vi "Actor Core.vi"(8 "error in":errorcluster, 11 "MakePrintTable in":refnum<class "MakePrintTable.lvclass">) -> (0 "error out":errorcluster, 3 "Actor out":refnum<class "Actor.lvclass">)   [LabVIEW 2015, in "ActorManagement.lvlib" / "MakePrintTable.lvclass"]
doc: "(<B>Filename</B>: Actor Framework.lvlib:Actor.lvclass:Actor Core.vi)\n\nReceives messages to the actor, reacts to them, and initiates any error handling that may shut the actor down.\n\nDescendant classes may override this VI to append parallel tasks for the actor to complete while it handles messages. Overrides use the Call Parent Method node."
uses:
  MakePrintTable.lvclass
  <vilib>/ActorFramework/Actor/Actor.lvclass
  <vilib>/ActorFramework/Actor/Actor.lvclass/Actor.ctl
  <vilib>/ActorFramework/Message Enqueuer/Message Enqueuer.lvclass/Message Enqueuer.ctl
  <vilib>/ActorFramework/Stop Msg/Stop Msg.lvclass/Stop Msg.ctl
  <vilib>/ActorFramework/Message Enqueuer/Init from Existing Queue.vi
  <vilib>/ActorFramework/Message Enqueuer/Enqueue Critical.vi
  <vilib>/ActorFramework/Message Priority Queue/Priority Enqueue.vi
  PluginWithDatabase/PluginWithDatabase.lvclass
  <vilib>/ActorFramework/Message Enqueuer/Message Enqueuer.lvclass
  <vilib>/ActorFramework/Stop Msg/Stop Msg.lvclass
panel:
  in  "Tab Control":enum32{"管理本周出勤"}(tab)
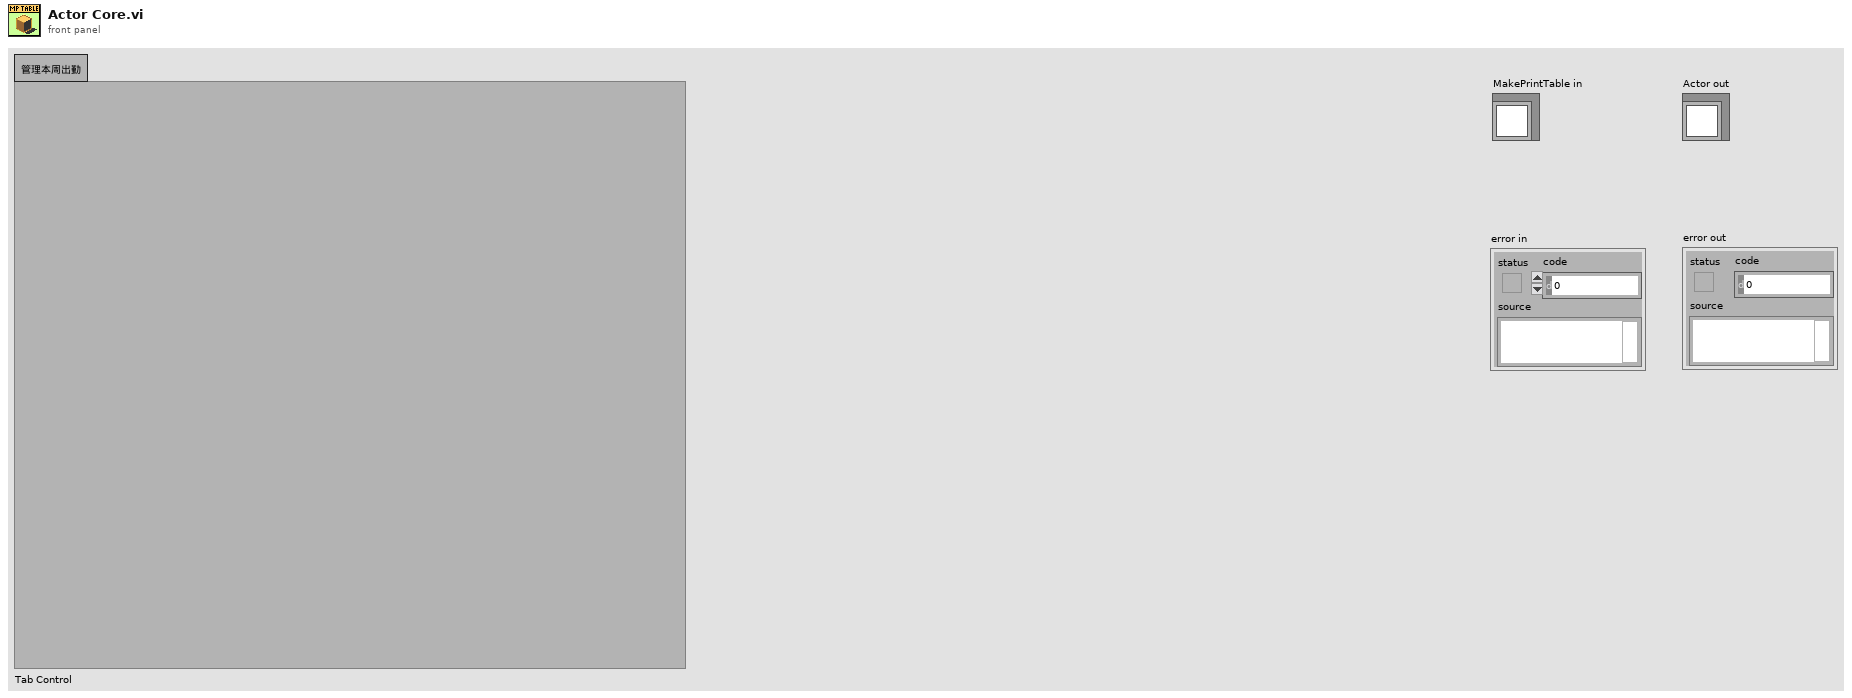
[diagram p1: front panel]
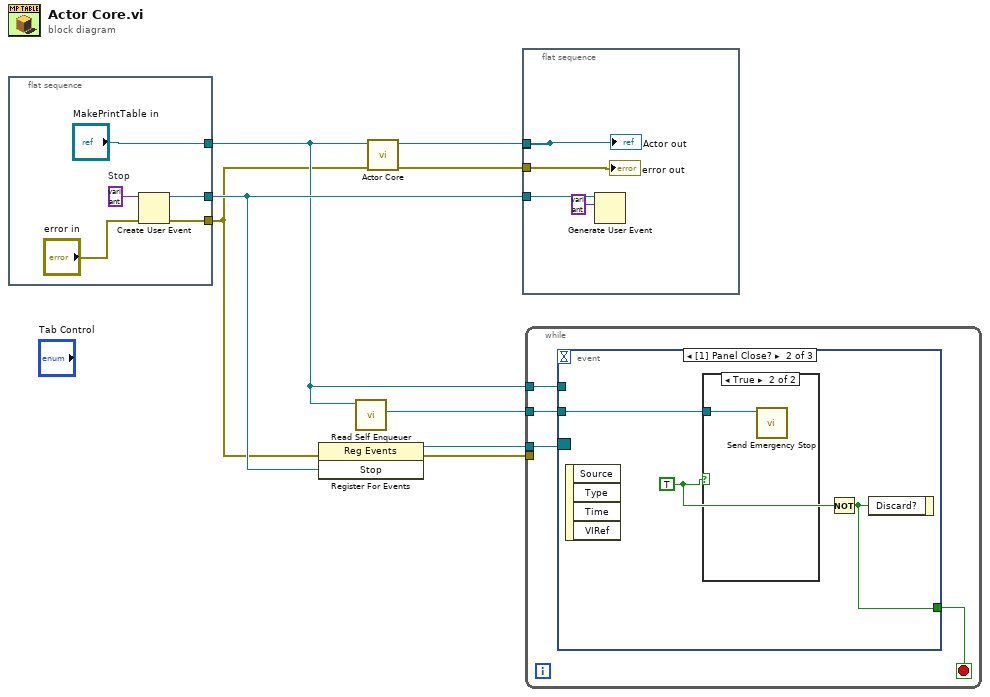
[diagram p0: block diagram]
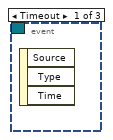
[diagram p2: hidden frame]
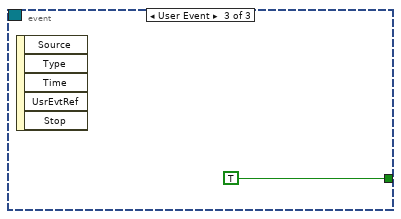
[diagram p4: hidden frame]
diagram:
  n1 = flat-sequence {
    tunnel: [w12] -> w5
    tunnel: [w11] -> w1
    tunnel: ["MakePrintTable in"] -> w4
    frame #0 {
      w13 = variant  # Stop
      n2 = Create User Event(user event datatype=w13, error in="error in") -> (user event=w12:refnum<user-event>, error out=w11:errorcluster)
    }
  }
  n3 = register-events(error in=w1, w5) -> (reference out=w6:refnum<event-registration>, error out=w7:errorcluster)  [unwired: 1 in]
  n4 = call <vilib>:"Read Self Enqueuer.vi"("Actor"=w4) -> ("Self Enqueuer"=w8:refnum<class "Message Enqueuer.lvclass">)  [unwired: 10 in]
  n5 = call-parent "Actor Core.vi"("error in"=w1, "Actor in"=w4) -> ("error out"=w2:errorcluster, "Actor out"=w3:refnum<class "Actor.lvclass">)  [unwired: 8 in]
  n6 = flat-sequence {
    tunnel: w5 -> [w17]
    tunnel: [w15] -> _
    tunnel: w3 -> [w15]
    tunnel: w2 -> [w14]
    frame #0 {
      n7 = Generate User Event(user event=w17, event data cluster=variant ("event data")) -> ()  [unwired: 2 in, 2 out]
      "error out" <- w14
      "Actor out" <- w15
    }
  }
  n8 = while {
    tunnel: w6 -> [w21]
    tunnel: w7 -> [_]
    tunnel: w8 -> [w20]
    tunnel: w4 -> [w19]
    stop <- w18 stop-if-true
    n9 = event shown="[1] Panel Close?" {
      selector: w21 -> [_ _ _]
      dyn-events: _ -> [_ _ _]
      timeout: _ -> [_ _ _]
      tunnel: w20 -> [_ w24 _]
      tunnel: w19 -> [_ _ _]
      tunnel: [_ w22 TRUE] -> w18
      event Timeout {
        n10 = event-data() -> ()  [unwired: 1 in, 3 out]
      }
      event Panel Close? {
        w23 = TRUE
        n11 = event-data() -> ()  [unwired: 1 in, 4 out]
        n12 = case shown="True" w23 {
          tunnel: w24 -> [_ w25]
          frame False {
          }
          frame True {
            n13 = call <vilib>:"Send Emergency Stop.vi"("Message Enqueuer"=w25) -> ()  [unwired: 10 in, 1 out]
          }
        }
        n14 = Not(x=w23) -> (.not. x?=w22:bool)
        n15 = event-data("Discard?"=w22) -> ()  [unwired: 1 in, 1 out]
      }
      event User Event {
        n16 = event-data() -> ()  [unwired: 1 in, 5 out]
      }
    }
  }
